vi "Leitura AnaA0.vi"(8 "error in (no error)":errorcluster, 11 "VISA Refnum in":refnum<visa-resource-name>) -> (0 "error out":errorcluster, 2 "Gauge":dbl(knob), 3 "VISA Refnum out":refnum<visa-resource-name>)   [LabVIEW 2018]
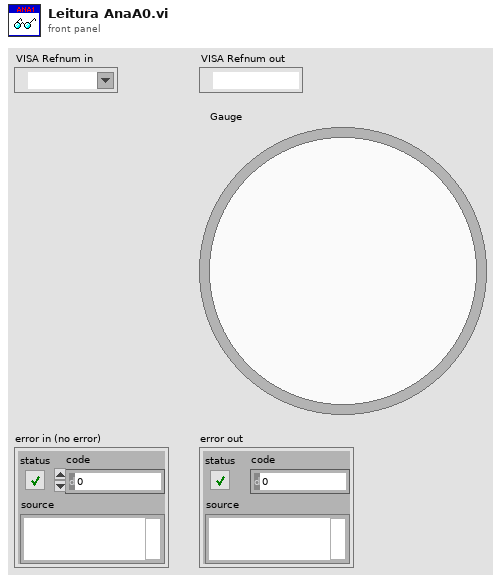
[diagram p1: front panel]
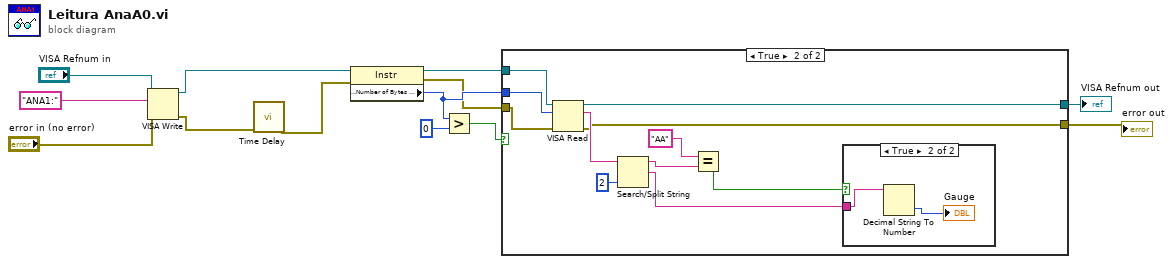
[diagram p0: block diagram]
diagram:
  n1 = VISA Write(VISA resource name="VISA Refnum in", write buffer="ANA1:", error in (no error)="error in (no error)") -> (VISA resource name out=w4:refnum<visa-resource-name>, error out=w2:errorcluster)  [unwired: 1 out]
  n2 = call "Time Delay"("error in (no error)"=w2) -> ("error out"=w3:errorcluster)  [unwired: 10 in]
  n3 = property class="Instr"(reference=w4, error in=w3) -> (reference out=w7:refnum<visa-resource-name>, error out=w8:errorcluster, "Serial Settings:Number of Bytes at Serial Port"=w9:u32)
  n4 = Greater?(x=w9, y=u32 0) -> (0:w6:bool)
  n5 = case shown="True" w6 {
    tunnel: w7 -> [w15 w26]
    tunnel: w8 -> [w14 w25]
    tunnel: w9 -> [_ w24]
    tunnel: [w15 w17] -> w12
    tunnel: [w14 w16] -> w13
    frame False {
    }
    frame True {
      n6 = VISA Read(VISA resource name=w26, byte count=w24, error in (no error)=w25) -> (VISA resource name out=w17:refnum<visa-resource-name>, read buffer=w22:string, error out=w16:errorcluster)  [unwired: 1 out]
      n7 = Search/Split String(string=w22, offset (0)=2) -> (substring before match=w21:string, match + rest of string=w18:string)  [unwired: 1 in, 1 out]
      n8 = Equal?(x="AA", y=w21) -> (x = y?=w19:bool)
      n9 = case shown="True" w19 {
        tunnel: w18 -> [_ w28]
        frame False {
        }
        frame True {
          n10 = Decimal String To Number(string=w28) -> (number=→"Gauge":i32)  [unwired: 2 in, 1 out]
        }
      }
    }
  }
  "VISA Refnum out" <- w12
  "error out" <- w13
